vi "diff.vi"   [LabVIEW 2015]
doc: "Calculates the difference between the neighbouring elements of the array"
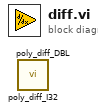
[diagram p0: block diagram]
diagram:
  n1 = call "poly_diff_I32.vi"() -> ()  [unwired: 9 in, 1 out]
  n2 = call "poly_diff_DBL.vi"() -> ()  [unwired: 9 in, 1 out]
